vi "实时数据发送间隔全局.vi"() -> ()   [LabVIEW 2016]
panel:
  in  "实时数据发送间隔":u32
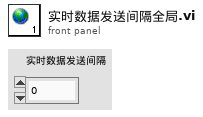
[diagram p1: front panel]
diagram:
